vi "set_relay.vi"(1 "Slot":i32=10 min=0 max=14, 2 "Relay":i32=1 min=1 max=12, 3 "Relay Status":bool) -> ()   [LabVIEW 2011]
uses:
  globals.vi
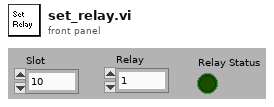
[diagram p1: front panel]
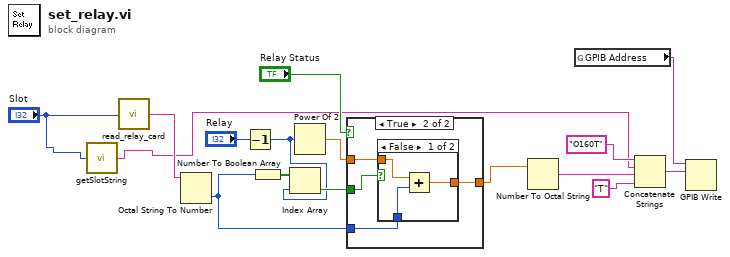
[diagram p0: block diagram]
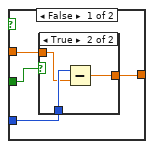
[diagram p2: hidden frame]
diagram:
  n1 = call "getSlotString.vi"("Slot"="Slot") -> ("string"=w1:string)
  n2 = call "read_relay_card.vi"("Slot"="Slot") -> ("data"=w16:string)
  n3 = Octal String To Number(4:w16) -> (0:w6:u32)  [unwired: 3 out]
  n4 = Decrement(x="Relay") -> (x-1=w8:i32)
  n5 = Number To Boolean Array(number=w6) -> (Boolean array=w12:bool[])
  n6 = Index Array(array=w12, index=w8) -> (element=w11:bool)
  n7 = Power Of 2(x=w8) -> (2^x=w9:dbl)
  n8 = case shown="True" "Relay Status" {
    tunnel: w11 -> [w17 w28]
    tunnel: w6 -> [w18 w27]
    tunnel: w9 -> [w19 w26]
    tunnel: [w20 w25] -> w10
    frame False {
      n9 = case shown="True" w17 {
        tunnel: w18 -> [w21 w23]
        tunnel: w19 -> [_ w22]
        tunnel: [w21 w24] -> w20
        frame False {
        }
        frame True {
          n10 = Subtract(x=w23, y=w22) -> (x-y=w24:dbl)
        }
      }
    }
    frame True {
      n11 = case shown="False" w28 {
        tunnel: w27 -> [w31 w32]
        tunnel: w26 -> [w30 _]
        tunnel: [w29 w32] -> w25
        frame False {
          n12 = Add(x=w30, y=w31) -> (x+y=w29:dbl)
        }
        frame True {
        }
      }
    }
  }
  n13 = Number To Octal String(2:w10) -> (0:w5:string)  [unwired: 1 out]
  n14 = global read "globals.vi" "GPIB Address"() -> (w15:string)
  n15 = Concatenate Strings("O160T", w1, w5, "T" ("string")) -> (w7:string)
  n16 = GPIB Write(0:w15, 1:w7) -> ()  [unwired: 1 in, 4 out]
